vi "战斗进度条.vi"() -> ()   [LabVIEW 2013]
panel:
  in  "停止":bool
  in  "怪物速度":i32
  in  "数值":i32
  out "滑动杆 2":u8(slide) scale=0.0..100.0
  out "滑动杆":u8(slide) scale=0.0..100.0
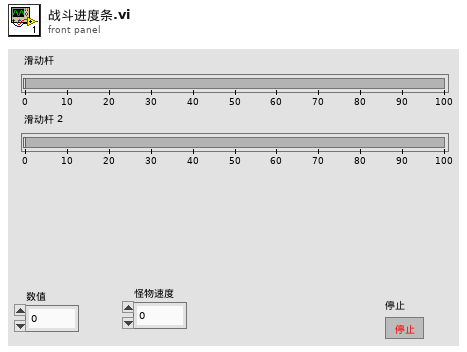
[diagram p1: front panel]
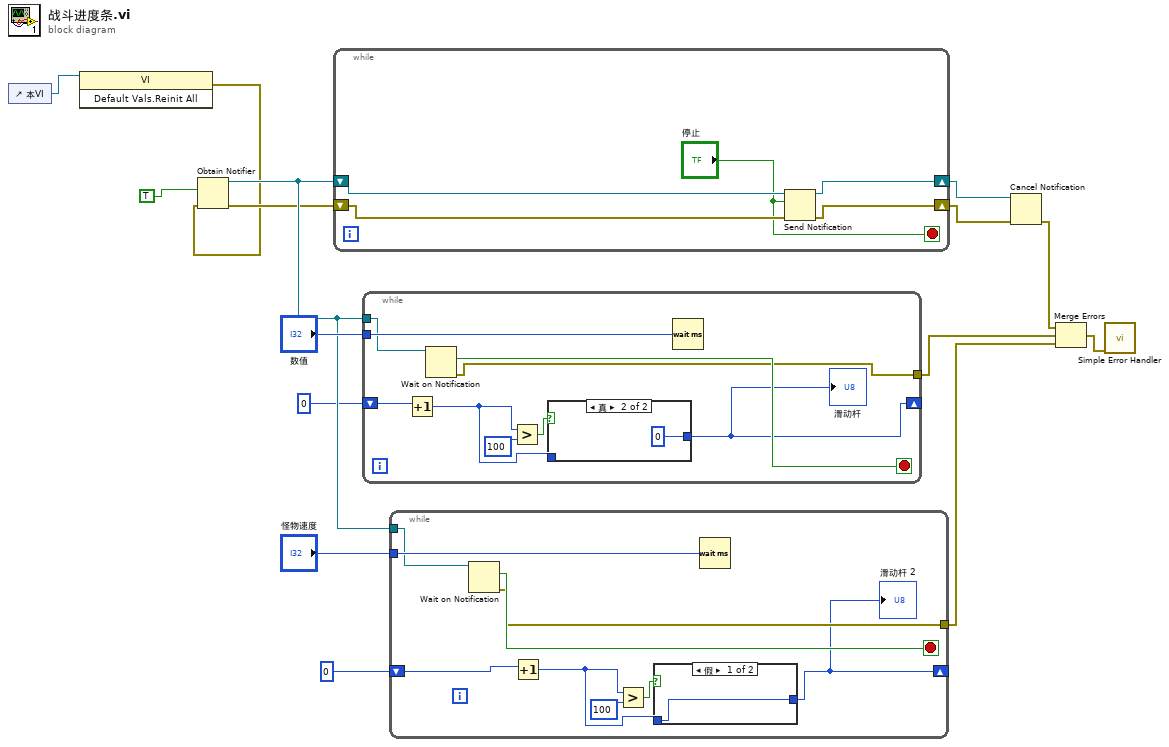
[diagram p0: block diagram]
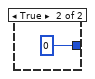
[diagram p2: hidden frame]
diagram:
  n1 = control-ref of="本VI"() -> (w2:refnum<vi>)
  n2 = invoke class="VI" method="Default Vals.Reinit All"(reference=w2) -> (error out=w1:errorcluster)  [unwired: 2 in, 2 out]
  n3 = Obtain Notifier(notification data type=TRUE, error in (no error)=w1) -> (notifier out=w12:refnum<notifier>, error out=w11:errorcluster)  [unwired: 2 in, 1 out]
  n4 = while {
    shift-right: [w17] -> w10
    shift-left: w12 -> [w20]
    shift-right: [w16] -> w5
    shift-left: w11 -> [w19]
    stop <- "停止" stop-if-true
    n5 = Send Notification(notification="停止", notifier=w20, error in (no error)=w19) -> (notifier out=w17:refnum<notifier>, error out=w16:errorcluster)
  }
  n6 = while {
    tunnel: "数值" -> [w29]
    tunnel: w12 -> [w28]
    tunnel: [w26] -> w8
    shift-right: [w21] -> _
    shift-left: 0 -> [w23]
    stop <- w27 stop-if-true
    n7 = Increment(x=w23) -> (x+1=w22:i32)
    n8 = Wait on Notification(notifier=w28) -> (notification=w27:bool, error out=w26:errorcluster)  [unwired: 3 in, 2 out]
    n9 = Greater?(x=w22, y=100) -> (0:w24:bool)
    n10 = case shown="真" w24 {
      tunnel: [w30 0] -> w21
      tunnel: w22 -> [w30 _]
      frame False {
      }
      frame True {
      }
    }
    "滑动杆" <- w21
    n11 = Wait (ms)(milliseconds to wait=w29) -> ()  [unwired: 1 out]
  }
  n12 = while {
    tunnel: "怪物速度" -> [w40]
    tunnel: w12 -> [w39]
    tunnel: [w37] -> w7
    shift-right: [w32] -> _
    shift-left: 0 -> [w33]
    stop <- w38 stop-if-true
    n13 = Wait on Notification(notifier=w39) -> (notification=w38:bool, error out=w37:errorcluster)  [unwired: 3 in, 2 out]
    n14 = Increment(x=w33) -> (x+1=w34:i32)
    n15 = Greater?(x=w34, y=100) -> (0:w35:bool)
    n16 = case shown="假" w35 {
      tunnel: [w41 0] -> w32
      tunnel: w34 -> [w41 _]
      frame False {
      }
      frame True {
      }
    }
    "滑动杆 2" <- w32
    n17 = Wait (ms)(milliseconds to wait=w40) -> ()  [unwired: 1 out]
  }
  n18 = Cancel Notification(0:w10, 3:w5) -> (11:w9:errorcluster)  [unwired: 2 out]
  n19 = Merge Errors(w9, w8, w7) -> (w6:errorcluster)
  n20 = call <vilib>:"Simple Error Handler.vi"("error in (no error)"=w6) -> ()  [unwired: 4 in, 5 out]
